vi "Open Butterfly Talon SRX.vi"(7 "CAN Talon SRX Ref":T1, 8 "error in (no error)":errorcluster, 9 "Cluster":T6, 10 "secondsFromNeutralToFull":dbl, 11 "Motor Control Neutral Mode":T7) -> (0 "error out":errorcluster, 2 "PhoenixMotorControlDevRef":T1, 3 "PhoenixMotorControlDevRef 2":T1)   [LabVIEW 2018]
uses:
  <vilib>/Rock Robotics/WPI/ThirdParty/Phoenix-LabVIEW/Motor Controller/Controls/CTRE_Phoenix_MotorControl_NeutralMode.ctl
  <vilib>/Rock Robotics/WPI/MotorControl/WPI_MotorControlDeviceRef.ctl
  <vilib>/Rock Robotics/WPI/MotorControl/WPI_MotorControlType.ctl
  <vilib>/Rock Robotics/SystemInterfaces/DIO/FPGA_DIOPWMChannel.ctl
  <vilib>/Rock Robotics/WPI/PWM/WPI_PWMDeadband.ctl
  <vilib>/Rock Robotics/SystemInterfaces/DIO/FPGA_DIOChannel.ctl
panel:
  out "PhoenixMotorControlDevRef 3":T1
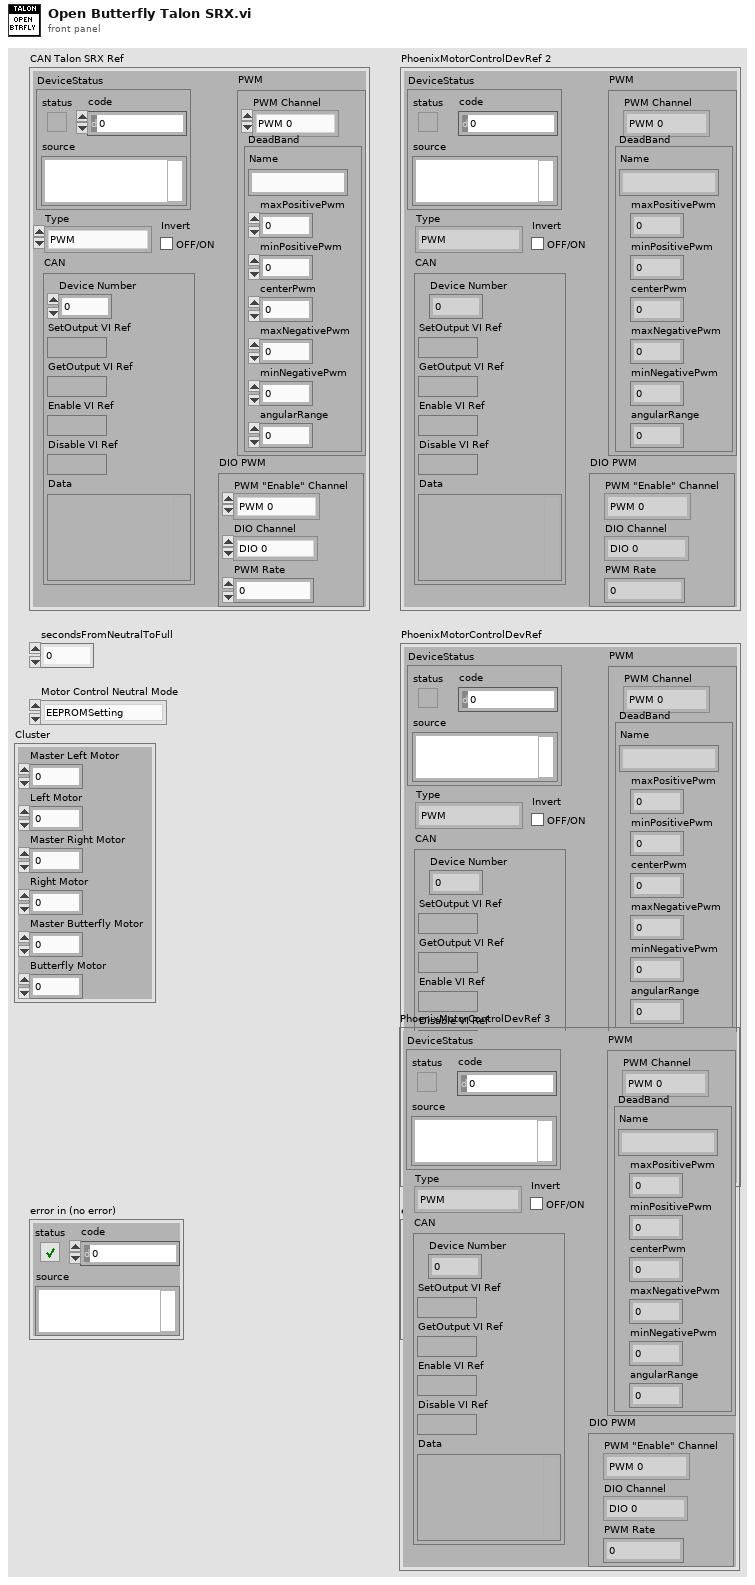
[diagram p1: front panel]
types:
  T1 = typedef "WPI_MotorControlDeviceRef.ctl" = cluster{"DeviceStatus":errorcluster, "Type":T2, "PWM":cluster{"PWM Channel":T3, "DeadBand":T4}, "CAN":cluster{"Device Number":u8, "SetOutput VI Ref":variant, "GetOutput VI Ref":variant, "Enable VI Ref":variant, "Disable VI Ref":variant, "Data":variant}, "Invert":bool, "DIO PWM":cluster{"PWM \"Enable\" Channel":T3, "DIOChannel":T5, "PWM Rate":dbl}}
  T2 = typedef "WPI_MotorControlType.ctl" = enum16{"PWM", "CAN", "DIO PWM"}
  T3 = typedef "FPGA_DIOPWMChannel.ctl" = enum8{"PWM 0", "PWM 1", "PWM 2", "PWM 3", "PWM 4", "PWM 5", "PWM 6", "PWM 7", "PWM 8", "PWM 9", "PWM MXP 0", "PWM MXP 1", "PWM MXP 2", "PWM MXP 3", "PWM MXP 4", "PWM MXP 5", "PWM MXP 6", "PWM MXP 7", "PWM MXP 8", "PWM MXP 9", "Invalid"}
  T4 = typedef "WPI_PWMDeadband.ctl" = cluster{"Name":string, "maxPositivePwm":i32, "minPositivePwm":i32, "centerPwm":i32, "maxNegativePwm":i32, "minNegativePwm":i32, "angularRange":u16}
  T5 = typedef "FPGA_DIOChannel.ctl" = enum8{"DIO 0", "DIO 1", "DIO 2", "DIO 3", "DIO 4", "DIO 5", "DIO 6", "DIO 7", "DIO 8", "DIO 9", "DIO MXP 0", "DIO MXP 1", "DIO MXP 2", "DIO MXP 3", "DIO MXP 4", "DIO MXP 5", "DIO MXP 6", "DIO MXP 7", "DIO MXP 8", "DIO MXP 9", "DIO MXP 10", "DIO MXP 11", "DIO MXP 12", "DIO MXP 13", "DIO MXP 14", "DIO MXP 15", "SPI Port CS1", "SPI Port CS2", "SPI Port CS3", "SPI Port MISO", "SPI Port MOSI", "Invalid"}
  T6 = cluster{"Master Left Motor":u8, "Left Motor":u8, "Master Right Motor":u8, "Right Motor":u8, "Master Butterfly Motor":i32, "Butterfly Motor":i32}
  T7 = typedef "CTRE_Phoenix_MotorControl_NeutralMode.ctl" = enum8{"EEPROMSetting", "Override to Coast", "Override to Brake"}
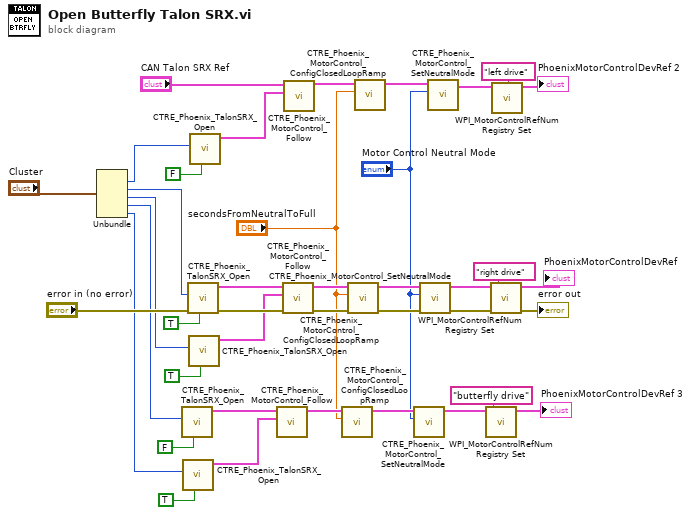
[diagram p0: block diagram]
diagram:
  n1 = Unbundle("Cluster") -> ("Left Motor"=w27:u8, "Master Right Motor"=w26:u8, "Right Motor"=w25:u8, "Master Butterfly Motor"=w13:i32, "Butterfly Motor"=w14:i32)  [unwired: 1 out]
  n2 = call <vilib>:"CTRE_Phoenix_TalonSRX_Open.vi"("Invert"=FALSE, "Device Number"=w13) -> ("CAN Talon SRX Ref"=w16:T1)  [unwired: 8 in, 1 out]
  n3 = call <vilib>:"CTRE_Phoenix_TalonSRX_Open.vi"("Invert"=TRUE, "Device Number"=w14) -> ("CAN Talon SRX Ref"=w15:T1)  [unwired: 8 in, 1 out]
  n4 = call <vilib>:"CTRE_Phoenix_TalonSRX_Open.vi"("Invert"=TRUE, "error in"="error in (no error)", "Device Number"=w26) -> ("error out"=w33:errorcluster, "CAN Talon SRX Ref"=w32:T1)  [unwired: 7 in]
  n5 = call <vilib>:"CTRE_Phoenix_TalonSRX_Open.vi"("Invert"=TRUE, "Device Number"=w25) -> ("CAN Talon SRX Ref"=w31:T1)  [unwired: 8 in, 1 out]
  n6 = call <vilib>:"CTRE_Phoenix_TalonSRX_Open.vi"("Invert"=FALSE, "Device Number"=w27) -> ("CAN Talon SRX Ref"=w28:T1)  [unwired: 8 in, 1 out]
  n7 = call <vilib>:"CTRE_Phoenix_MotorControl_Follow.vi"("Master Controller to Follow"=w15, "PhoenixMotorControlDevRef"=w16) -> ("PhoenixMotorControlDevRef"=w23:T1)  [unwired: 8 in, 1 out]
  n8 = call <vilib>:"CTRE_Phoenix_MotorControl_Follow.vi"("error in (no error)"=w33, "Master Controller to Follow"=w31, "PhoenixMotorControlDevRef"=w32) -> ("error out"=w11:errorcluster, "PhoenixMotorControlDevRef"=w40:T1)  [unwired: 7 in]
  n9 = call <vilib>:"CTRE_Phoenix_MotorControl_Follow.vi"("Master Controller to Follow"=w28, "PhoenixMotorControlDevRef"="CAN Talon SRX Ref") -> ("PhoenixMotorControlDevRef"=w38:T1)  [unwired: 8 in, 1 out]
  n10 = call <vilib>:"CTRE_Phoenix_MotorControl_ConfigClosedLoopRamp.vi"("secondsFromNeutralToFull"="secondsFromNeutralToFull", "PhoenixMotorControlDevRef"=w23) -> ("PhoenixMotorControlDevRef"=w22:T1)  [unwired: 8 in, 1 out]
  n11 = call <vilib>:"CTRE_Phoenix_MotorControl_ConfigClosedLoopRamp.vi"("error in (no error)"=w11, "secondsFromNeutralToFull"="secondsFromNeutralToFull", "PhoenixMotorControlDevRef"=w40) -> ("error out"=w12:errorcluster, "PhoenixMotorControlDevRef"=w39:T1)  [unwired: 7 in]
  n12 = call <vilib>:"CTRE_Phoenix_MotorControl_ConfigClosedLoopRamp.vi"("secondsFromNeutralToFull"="secondsFromNeutralToFull", "PhoenixMotorControlDevRef"=w38) -> ("PhoenixMotorControlDevRef"=w37:T1)  [unwired: 8 in, 1 out]
  n13 = call <vilib>:"CTRE_Phoenix_MotorControl_SetNeutralMode.vi"("Motor Control Neutral Mode"="Motor Control Neutral Mode", "PhoenixMotorControlDevRef"=w22) -> ("PhoenixMotorControlDevRef"=w21:T1)  [unwired: 8 in, 1 out]
  n14 = call <vilib>:"CTRE_Phoenix_MotorControl_SetNeutralMode.vi"("error in (no error)"=w12, "Motor Control Neutral Mode"="Motor Control Neutral Mode", "PhoenixMotorControlDevRef"=w39) -> ("error out"=w10:errorcluster, "PhoenixMotorControlDevRef"=w9:T1)  [unwired: 7 in]
  n15 = call <vilib>:"CTRE_Phoenix_MotorControl_SetNeutralMode.vi"("Motor Control Neutral Mode"="Motor Control Neutral Mode", "PhoenixMotorControlDevRef"=w37) -> ("PhoenixMotorControlDevRef"=w4:T1)  [unwired: 8 in, 1 out]
  n16 = call <vilib>:"WPI_MotorControlRefNum Registry Set.vi"("refnum name"="butterfly drive", "MotorControlDevRef"=w21) -> ("MotorControlDevRef"=→"PhoenixMotorControlDevRef 3":T1)  [unwired: 8 in, 1 out]
  n17 = call <vilib>:"WPI_MotorControlRefNum Registry Set.vi"("error in (no error)"=w10, "refnum name"="right drive", "MotorControlDevRef"=w9) -> ("error out"=→"error out":errorcluster, "MotorControlDevRef"=→"PhoenixMotorControlDevRef":T1)  [unwired: 7 in]
  n18 = call <vilib>:"WPI_MotorControlRefNum Registry Set.vi"("refnum name"="left drive", "MotorControlDevRef"=w4) -> ("MotorControlDevRef"=→"PhoenixMotorControlDevRef 2":T1)  [unwired: 8 in, 1 out]
